vi "H5Aread (Variant).vi"(4 "Data":variant, 6 "error in (no error)":errorcluster, 8 "HDF5 Type Ref (match data)":T1, 9 "HDF5 Attr Ref":T1) -> (0 "error out":errorcluster, 2 "Data out":variant, 3 "HDF5 Attr Ref out":T1)   [LabVIEW 2017]
doc: "Reads an attribute."
uses:
  <vilib>/UPVI/lvhdf5/library.llb/HDF5 Ref.ctl
  <vilib>/UPVI/lvhdf5/identifier.llb/H5Iget_type.vi
  <vilib>/UPVI/lvhdf5/h5helper.dll
panel:
  # "LVHDF5 Toolkit\nCopyright (c) 2005-2013 by Jason D. Sommerville\nCopyright (c) 2014 by UPVI, LLC.\n\nThis use and distribution of this file is governed by the terms found in \nLICENSE.txt distributed with this toolkit and installed at\n <user.lib>\\_lvhdf5\\LICENSE.txt"
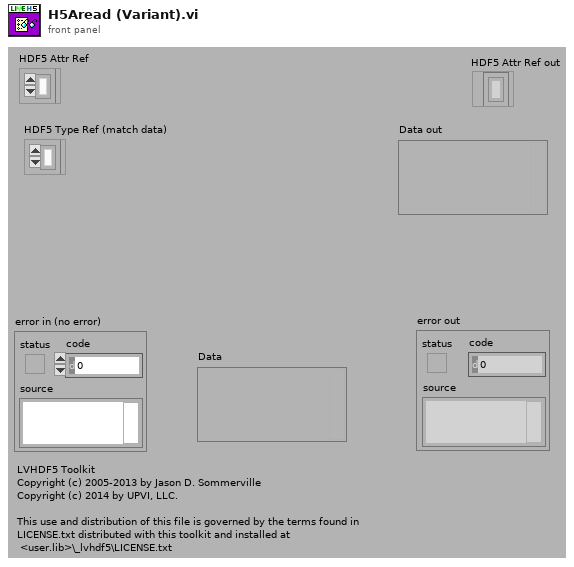
[diagram p1: front panel]
types:
  T1 = typedef "HDF5 Ref.ctl" = refnum<k1>
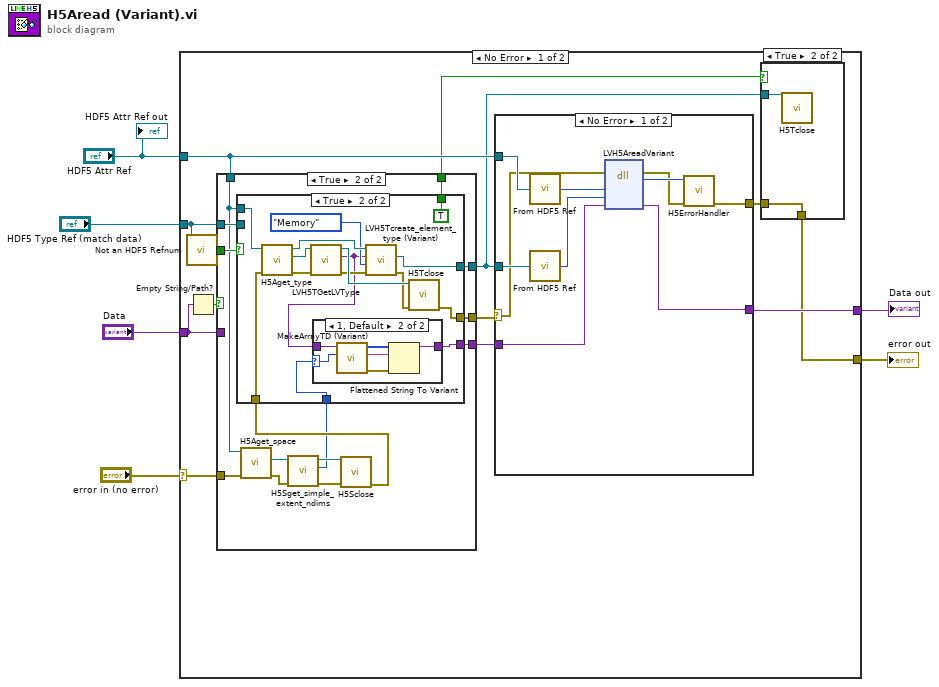
[diagram p0: block diagram]
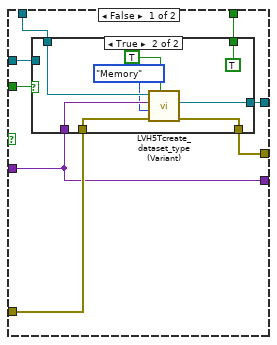
[diagram p2: hidden frame]
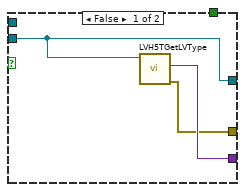
[diagram p4: hidden frame]
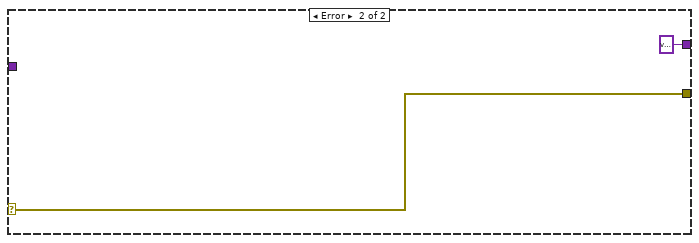
[diagram p8: hidden frame]
diagram:
  n1 = case shown="No Error" "error in (no error)" {
    selector: "error in (no error)" -> [w17 w92]
    tunnel: [w10 w92] -> w5
    tunnel: "HDF5 Attr Ref" -> [w18 _]
    tunnel: [w19 variant ("Variant")] -> w2
    tunnel: "Data" -> [w14 _]
    tunnel: "HDF5 Type Ref (match data)" -> [w12 _]
    frame No Error {
      n2 = call <vilib>:"Not an HDF5 Refnum.vi"("HDF5 Ref"=w12) -> ("Not an HDF5 Refnum"=w11:bool)
      n3 = Empty String/Path?(string/path=w14) -> (empty?=w13:bool)
      n4 = case shown="True" w13 {
        tunnel: w14 -> [w20 _]
        tunnel: w18 -> [w27 w46]
        tunnel: w17 -> [w26 w45]
        tunnel: [w24 w48] -> w16
        tunnel: [w23 w49] -> w15
        tunnel: w12 -> [w22 w50]
        tunnel: w11 -> [w21 w51]
        tunnel: [w20 w47] -> w8
        tunnel: [w25 w38] -> w7
        frame False {
          n5 = case shown="True" w21 {
            tunnel: w20 -> [_ w37]
            tunnel: w27 -> [_ w36]
            tunnel: [w28 w34] -> w23
            tunnel: w26 -> [w29 w33]
            tunnel: [w29 w32] -> w25
            tunnel: [_ TRUE] -> w24
            tunnel: w22 -> [w28 _]
            frame False {
            }
            frame True {
              n6 = call <vilib>:"LVH5Tcreate_dataset_type (Variant).vi"("Don't use cache"=TRUE, "error in (no error)"=w33, "Type"=enum16{"File", "Memory"}."Memory", "Data"=w37, "HDF5 Ref"=w36) -> ("error out"=w32:errorcluster, "HDF5 Type Ref"=w34:T1)  [unwired: 2 in, 3 out]
            }
          }
        }
        frame True {
          n7 = call <vilib>:"H5Aget_space.vi"("error in (no error)"=w45, "HDF5 Attr Ref"=w46) -> ("error out"=w42:errorcluster, "HDF5 Dataspace Ref"=w44:T1)  [unwired: 5 in, 1 out]
          n8 = call <vilib>:"H5Sget_simple_extent_ndims.vi"("error in (no error)"=w42, "HDF5 Space Ref"=w44) -> ("error out"=w41:errorcluster, "Rank"=w39:i32, "HDF5 Ref out"=w43:T1)  [unwired: 5 in]
          n9 = call <vilib>:"H5Sclose.vi"("error in (no error)"=w41, "HDF5 Dataspace Ref"=w43) -> ("error out"=w40:errorcluster)  [unwired: 7 in]
          n10 = case shown="True" w51 {
            tunnel: w46 -> [_ w55]
            tunnel: w50 -> [w54 _]
            tunnel: [w52 w56] -> w38
            tunnel: [w54 w63] -> w49
            tunnel: [_ TRUE] -> w48
            tunnel: [w53 w57] -> w47
            tunnel: w40 -> [_ w60]
            tunnel: w39 -> [_ w59]
            frame False {
              n11 = call <vilib>:"LVH5TGetLVType.vi"("HDF5 Type Ref"=w54) -> ("error out"=w52:errorcluster, "Data Type"=w53:variant)  [unwired: 6 in, 3 out]
            }
            frame True {
              n12 = call <vilib>:"H5Aget_type.vi"("error in (no error)"=w60, "HDF5 Attr Ref"=w55) -> ("error out"=w66:errorcluster, "HDF5 Datatype Ref"=w65:T1, "HDF5 Attr Ref out"=w67:T1)  [unwired: 5 in]
              n13 = call <vilib>:"LVH5TGetLVType.vi"("error in (no error)"=w66, "HDF5 Type Ref"=w65) -> ("error out"=w68:errorcluster, "Data Type"=w58:variant, "HDF5 Type Ref out"=w69:T1)  [unwired: 5 in, 2 out]
              n14 = case shown="1, Default" w59 {
                selector: w59 -> [_ w76]
                tunnel: w58 -> [w70 w75]
                tunnel: [w70 w71] -> w57
                frame -1, 0 {
                }
                frame 1, Default {
                  n15 = call <vilib>:"MakeArrayTD (Variant).vi"("rank"=w76, "Element type_id"=w75) -> ("error out"=w74:errorcluster, "Default Data"=w73:string, "td"=w72:i16[])  [unwired: 7 in]
                  n16 = Flattened String To Variant(4:w74, 6:w73, 7:w72) -> (3:w71:variant)  [unwired: 1 out]
                }
              }
              n17 = call <vilib>:"LVH5Tcreate_element_type (Variant).vi"("error in (no error)"=w68, "Type"=enum16{"File", "Memory"}."Memory", "Data"=w58, "HDF5 Location Ref"=w67) -> ("error out"=w61:errorcluster, "HDF5 Type Ref"=w63:T1)  [unwired: 3 in, 3 out]
              n18 = call <vilib>:"H5Tclose.vi"("error in (no error)"=w61, "HDF5 Datatype Ref"=w69) -> ("error out"=w56:errorcluster)  [unwired: 7 in]
            }
          }
        }
      }
      n19 = case shown="No Error" w7 {
        selector: w7 -> [w83 w90]
        tunnel: [w88 _] -> w19
        tunnel: w18 -> [w87 _]
        tunnel: w15 -> [w86 _]
        tunnel: [w81 w90] -> w9
        tunnel: w8 -> [w80 _]
        frame No Error {
          n20 = call <vilib>:"From HDF5 Ref.vi"("HDF5 Ref"=w87) -> ("I32"=w89:i32)
          n21 = call <vilib>:"From HDF5 Ref.vi"("HDF5 Ref"=w86) -> ("I32"=w85:i32)
          n22 = dll-call lib="C:/Program Files/National Instruments/LabVIEW 2017/vi.lib/UPVI/lvhdf5/h5helper.dll" fn="LVH5AreadVariant"(error in=w83, "attr_id"=w89, "mem_type_id"=w85, "plvvar"=w80) -> (error out=w82:errorcluster, "return type"=w84:i32, "plvvar"=w88:variant)  [unwired: 4 in, 1 out]
          n23 = call <vilib>:"H5ErrorHandler.vi"("error in (no error)"=w82, "herr_t"=w84) -> ("error out"=w81:errorcluster)  [unwired: 3 in, 4 out]
        }
        frame Error {
        }
      }
      n24 = case shown="True" w16 {
        tunnel: w15 -> [_ w79]
        tunnel: [w77 w78] -> w10
        tunnel: w9 -> [w77 w78]
        frame False {
        }
        frame True {
          n25 = call <vilib>:"H5Tclose.vi"("HDF5 Datatype Ref"=w79) -> ()  [unwired: 8 in, 1 out]
        }
      }
    }
    frame Error {
    }
  }
  "error out" <- w5
  "Data out" <- w2
  "HDF5 Attr Ref out" <- "HDF5 Attr Ref"
